vi "Exercice Operations.vi"() -> ()   [LabVIEW 2018]
panel:
  in  "Dial":dbl(knob) max=9.0 scale=0.0..10.0
  out "Numeric 6":dbl
  out "Numeric 5":dbl
  out "Numeric 4":dbl
  out "Numeric 3":dbl
  in  "Numeric":dbl min=0.0 max=9.0
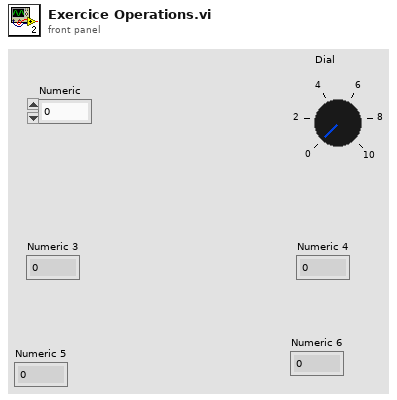
[diagram p1: front panel]
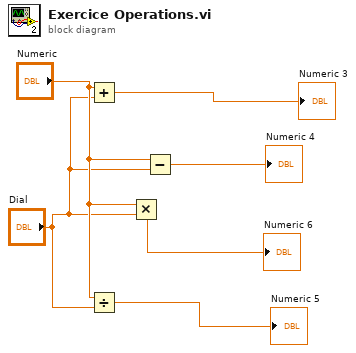
[diagram p0: block diagram]
diagram:
  n1 = Add(x="Numeric", y="Dial") -> (x+y=→"Numeric 3":dbl)
  n2 = Divide(x="Numeric", y="Dial") -> (x/y=→"Numeric 5":dbl)
  n3 = Multiply(x="Numeric", y="Dial") -> (x*y=→"Numeric 6":dbl)
  n4 = Subtract(x="Numeric", y="Dial") -> (x-y=→"Numeric 4":dbl)
